vi "newGUIHex.vi"() -> ()   [LabVIEW 2013]
uses:
  Controls/GUI_cluster.ctl
  Controls/eventtypdef1.ctl
  shared programs/GUI_Template/GUI_master/tcp_new_data_event.ctl
  shared programs/GUI_Template/GUI_master/tcp new data cluster.ctl
panel:
  in  "stepsize::7":dbl=0.02 caption="stepsize" min=0.0 max=10.0
  in  "uangle::7":dbl caption="u" min=-5.0 max=5.0
  in  "zpos::7":dbl=11.2 caption="z" min=-12.0 max=12.0
  in  "vangle::7":dbl caption="v" min=-5.0 max=5.0
  in  "ypos::7":dbl=4.0 caption="y" min=-20.0 max=20.0
  in  "wangle::7":dbl caption="w" min=-5.0 max=5.0
  in  "xpos::7":dbl=-1.0 caption="x" min=-20.0 max=20.0
  in  "<command>::7":bool
  out "GUIdevice 7":string="StagingHexapodPI"
  out "tcp data event":T1
  in  "GUI_cluster":T2={"Sub Panel"=refnum, "GUIdevice"="Bella_LP_Mode", "CtlRef"=refnum, "User Event in"=refnum}
  in  "stop":bool
  in  "stop 2":refnum<vi>
  in  "relativemove.ypos::7":bool
  in  "relativemove.xpos::7":bool
  in  "relativemove.yneg::7":bool
  in  "relativemove.xneg::7":bool
  in  "relativemove.zpos::7":bool
  in  "relativemove.zneg::7":bool
  in  "relativemove.wpos::7":bool
  in  "relativemove.upos::7":bool
  in  "relativemove.uneg::7":bool
  in  "relativemove.vpos::7":bool
  in  "relativemove.vneg::7":bool
  in  "relativemove.wneg::7":bool
  # "+Z"
  # "+Y"
  # "-X"
  # "+Y"
  # "+X"
  # "-Z"
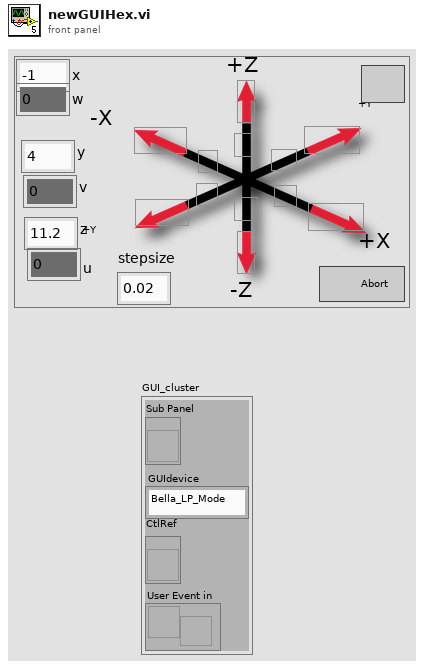
[diagram p1: front panel]
types:
  T1 = typedef "tcp_new_data_event.ctl" = refnum<user-event>
  T2 = typedef "GUI_cluster.ctl" = cluster{"Sub Panel":refnum<vi>, "GUIdevice":string, "CtlRef":refnum<vi>, "User Event in":refnum<user-event>}
  T3 = typedef "tcp new data cluster.ctl" = cluster{"EventEnum":enum16{"new data", "connection status update"}, "Device name":string}
  T4 = typedef "eventtypdef1.ctl" = cluster{"label":string, "Sub Panel":refnum<vi>, "CtlRef":refnum<vi>, "This VI":refnum<vi>}
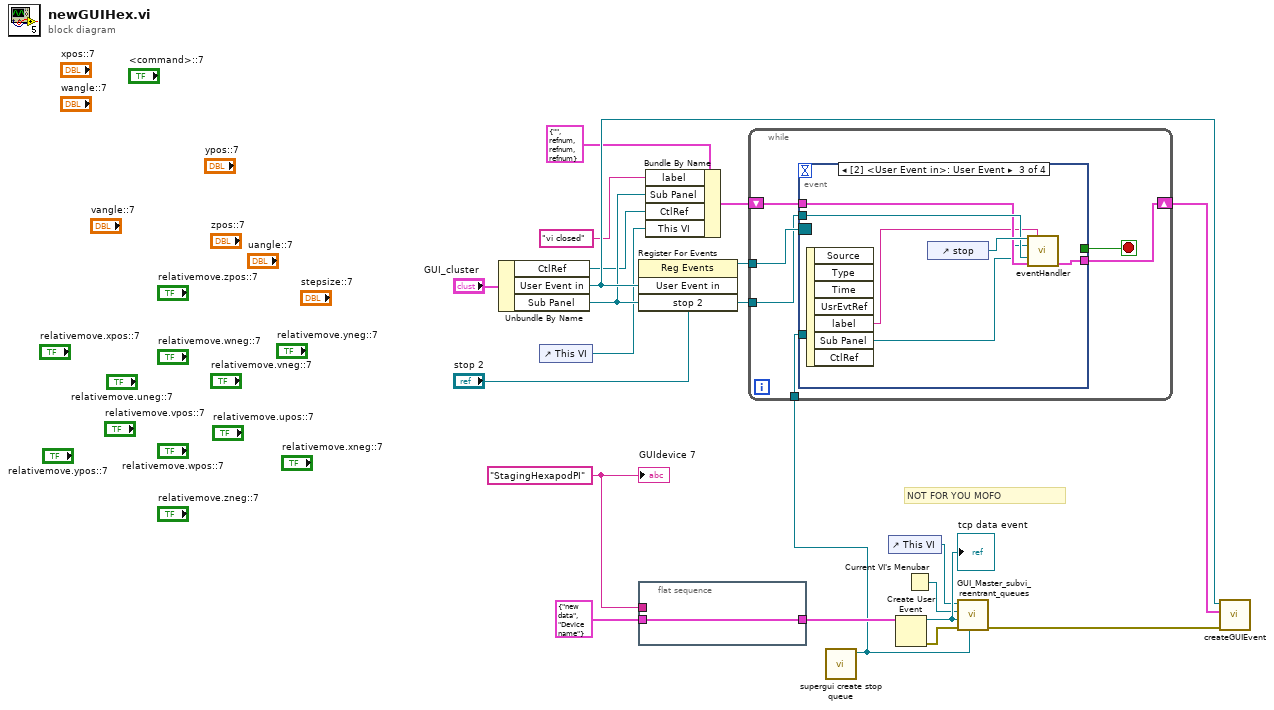
[diagram p0: block diagram]
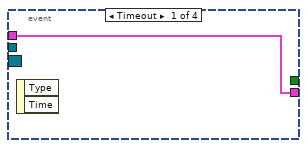
[diagram p2: hidden frame]
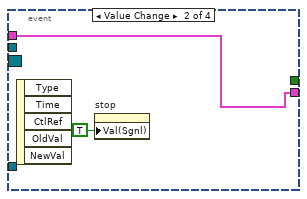
[diagram p3: hidden frame]
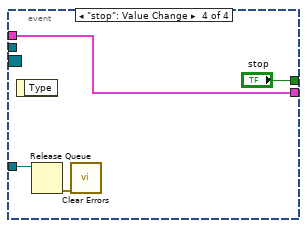
[diagram p4: hidden frame]
diagram:
  w12 = "StagingHexapodPI" ("GUIdevice")
  # "NOT FOR YOU MOFO"
  n1 = Unbundle By Name("GUI_cluster") -> ("CtlRef"=w10:refnum<vi>, "User Event in"=w17:refnum<user-event>, "Sub Panel"=w15:refnum<vi>)
  n2 = control-ref of="This VI"() -> (w11:refnum<vi>)
  n3 = register-events(w17, "stop 2") -> (reference out=w13:refnum<event-registration>)  [unwired: 2 in, 1 out]
  n4 = flat-sequence {
    tunnel: T3 {"EventEnum"=enum."new data", "Device name"="Device name"} ("New Event") -> [w21]
    tunnel: [w21] -> w9
    tunnel: w12 -> [_]
    frame #0 {
    }
  }
  n5 = Bundle By Name(cluster=T4 {"label"="", "Sub Panel"=refnum, "CtlRef"=refnum, "This VI"=refnum} ("event data"), "label"="vi closed", "Sub Panel"=w15, "CtlRef"=w10, "This VI"=w11) -> (w16:T4)
  n6 = call "supergui create stop queue.vi"() -> ("STOP Queue out"=w1:refnum<queue>)  [unwired: 11 in]
  n7 = while {
    tunnel: w13 -> [w27]
    tunnel: w15 -> [w25]
    shift-right: [w23] -> w19
    shift-left: w16 -> [w24]
    tunnel: w1 -> [w22]
    stop <- w26 stop-if-true
    n8 = event shown="[2] <User Event in>: User Event" {
      selector: w27 -> [_ _ _ _]
      dyn-events: _ -> [_ _ _ _]
      timeout: _ -> [_ _ _ _]
      tunnel: [_ _ _ "stop"] -> w26
      tunnel: w25 -> [_ _ w35 _]
      tunnel: w24 -> [w28 w30 w34 w39]
      tunnel: [w28 w30 w33 w39] -> w23
      tunnel: w22 -> [_ _ _ w38]
      event Timeout {
        n9 = event-data() -> ()  [unwired: 1 in, 2 out]
      }
      event Value Change {
        n10 = event-data() -> ()  [unwired: 1 in, 5 out]
        n11 = property on="stop" class="Bool (strict)"("Val(Sgnl)"=TRUE ("Value (Signaling)")) -> ()  [unwired: 2 in, 2 out]
      }
      event User Event {
        n12 = event-data() -> ("label"=w31:string, "Sub Panel"=w32:refnum<vi>)  [unwired: 1 in, 5 out]
        n13 = control-ref of="stop"() -> (w36:refnum<vi>)
        n14 = call "eventHandler.vi"("Boolean in"=w36, "label"=w31, "Sub Panel 2"=w32, "Sub Panel"=w35, "event data in"=w34) -> ("event data out"=w33:T4)  [unwired: 10 in]
      }
      event "stop": Value Change {
        n15 = event-data() -> ()  [unwired: 1 in, 1 out]
        n16 = Release Queue(queue=w38) -> (error out=w37:errorcluster)  [unwired: 2 in, 2 out]
        n17 = call <vilib>:"Clear Errors.vi"("error in (no error)"=w37) -> ()  [unwired: 6 in, 1 out]
      }
    }
  }
  n18 = control-ref of="This VI"() -> (w2:refnum<vi>)
  n19 = Create User Event(user event datatype=w9) -> (user event=w5:refnum<user-event>, error out=w4:errorcluster)  [unwired: 1 in]
  "tcp data event" <- w5
  n20 = Current VI's Menubar() -> (w3:refnum<k9>)
  n21 = call "GUI_Master_subvi_reentrant_queues.vi"("STOP Queue in"=w1, "error in (no error)"=w4, "tcp data event"=w5, "Caller menu reference"=w3, "Caller VI ref"=w2) -> ("error out"=w18:errorcluster)  [unwired: 6 in]
  n22 = call "createGUIEvent.vi"("error in (no error)"=w18, "event data"=w19, "User Event in"=w17) -> ()  [unwired: 8 in, 1 out]
  "GUIdevice 7" <- w12
